vi "Analog Output - 1 Channel - 1 Sample.vi"() -> ()   [LabVIEW 2019]
uses:
  <vilib>/myRIO/Instrument Drivers/Onboard IO/AO/typedefs/AO Reference.ctl
  <vilib>/myRIO/Common/Instrument Driver Framework/Utilities/typedefs/myRIO Generic Hardware Reference.ctl
  <vilib>/myRIO/Common/Instrument Driver Framework/Utilities/typedefs/Hardware Version Enum.ctl
  <vilib>/myRIO/Common/Instrument Driver Framework/Utilities/typedefs/myRIO v1.0 Reference.ctl
  <vilib>/myRIO/Common/Instrument Driver Framework/Utilities/typedefs/Generic FPGA Reference.ctl
  <vilib>/myRIO/Common/Instrument Driver Framework/myRIO v1.0/AO/typedefs/AO Channels List.ctl
  <vilib>/myRIO/Common/Instrument Driver Framework/myRIO v1.0/AO/typedefs/AO Channels Enum.ctl
  <vilib>/myRIO/Common/Instrument Driver Framework/Utilities/typedefs/Analog Scaling Constants List.ctl
  <vilib>/myRIO/Common/Instrument Driver Framework/Utilities/typedefs/Analog Scaling Constants.ctl
  <vilib>/userdefined/High Color/nirio_resource_hc.ctl
  <vilib>/myRIO/Common/Instrument Driver Framework/Utilities/vis/Is FPGA Ref Available.vi
  <vilib>/myRIO/Common/Instrument Driver Framework/ELVIS III v1.0/AO/vis/ELVIS III v1.1 Open AO.vi
  <vilib>/myRIO/Instrument Drivers/Onboard IO/AO/vis/Write.vi
  <vilib>/myRIO/Common/Instrument Driver Framework/Utilities/vis/Validate Channels.vi
  <vilib>/myRIO/Common/Instrument Driver Framework/ELVIS III v1.0/AO/vis/ELVIS III v1.0 Reserve AO.vi
  <vilib>/myRIO/Common/Instrument Driver Framework/myRIO v1.0/UART/vis/myRIO v1.0 Close UART.vi
  <vilib>/myRIO/Common/Instrument Driver Framework/ELVIS III v1.0/AO/vis/ELVIS III v1.0 Build MUX Configuration AO.vi
  <vilib>/Utility/VariantDataType/GetNumericInfo.vi
  <vilib>/Utility/error.llb/Error Cluster From Error Code.vi
  <vilib>/myRIO/Common/Instrument Driver Framework/ELVIS III v1.0/ELVIS III v1.1 Open.vi
  <vilib>/myRIO/Common/Instrument Driver Framework/ELVIS III v1.0/Resource Manager/vis/ELVIS III v1.0 Reserve Channel List.vi
  <vilib>/myRIO/Common/Instrument Driver Framework/myRIO v1.0/myRIO v1.0 Close.vi
  <vilib>/myRIO/Common/Instrument Driver Framework/ELVIS III v1.0/AO/vis/ELVIS III v1.0 Write AO.vi
  <vilib>/myRIO/Common/Instrument Driver Framework/Utilities/vis/FPGA Ref Manager.vi
  <vilib>/myRIO/Common/Instrument Driver Framework/ELVIS III v1.0/ELVIS III v1.0 Reset FPGA.vi
  <vilib>/myRIO/Common/Instrument Driver Framework/myRIO v1.0/IRQ/vis/myRIO v1.0 IRQ Info FGV.vi
  <vilib>/myRIO/Common/Instrument Driver Framework/myRIO v1.0/IRQ/vis/myRIO v1.0 Timer IRQ Info FGV.vi
  <vilib>/myRIO/Common/Instrument Driver Framework/myRIO v1.0/IRQ/vis/myRIO v1.0 ISR Agent.vi
  <vilib>/myRIO/Instrument Drivers/Utilities/vis/Reset Index.vi
  <vilib>/myRIO/Common/Instrument Driver Framework/myRIO v1.0/Resource Manager/vis/myRIO v1.0 Block Write Resource Manager.vi
  <vilib>/myRIO/Express VI/Onboard IO/AO/AO Express VI.xnode
  <vilib>/myRIO/Instrument Drivers/Onboard IO/AO/vis/myRIO AO Open.xnode
  <vilib>/myRIO/Instrument Drivers/Utilities/Utilities.lvlib
  <vilib>/myRIO/Instrument Drivers/Onboard IO/AO/AO.lvlib
panel:
  in  "A/AO0 (V)":dbl min=-10.0 max=10.0 step=0.1
  in  "Stop":bool
  # "ELVIS III Control IO"
  # "模拟输出单通道"
  # "Overview: Generates a voltage value on Bank A, Channel AO0 (A/AO0).\nInstructions:\n1. Select a voltage value below.\n2. Connect A/AO0 to the positive lead of the load, and connect AGND to the negative lead of the load. AGND is the ground reference terminal for analog output channels.\n3. Run the VI.\nNote: You can change the AO value while the VI is running."
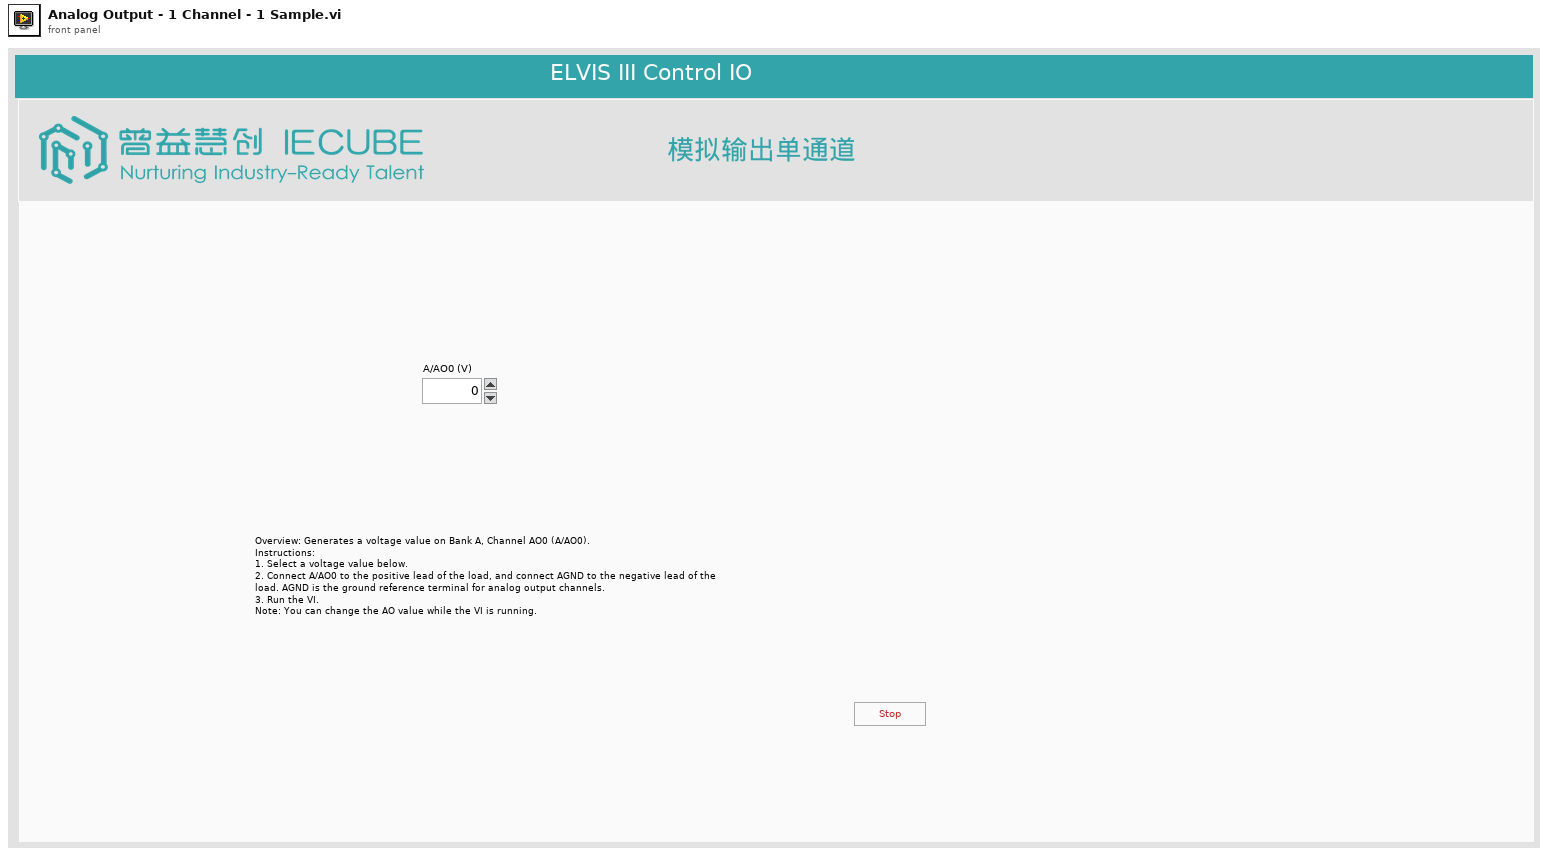
[diagram p1: front panel]
types:
  T1 = typedef "AO.lvlib/AO Reference.ctl" = cluster{"myRIO Reference":T2, "AO Channel List":T6, "AO Scaling Constant List":T8}
  T2 = typedef "myRIO Generic Hardware Reference.ctl" = cluster{"myRIO Model":T3, "myRIO Hardware Reference":T4}
  T3 = typedef "Hardware Version Enum.ctl" = enum16{"Unknown", "myRIO-1900", "myRIO-1950", "roboRIO", "NI ELVIS RIO CM", "ELVIS III"}
  T4 = typedef "myRIO v1.0 Reference.ctl" = cluster{"Generic FPGA Reference":T5, "Allow multiple opens":bool}
  T5 = typedef "Generic FPGA Reference.ctl" = refnum<k20>
  T6 = typedef "AO Channels List.ctl" = T7[]
  T7 = typedef "AO Channels Enum.ctl" = enum16{"Not Connected", "AudioOut/Left", "AudioOut/Right", "C/AO0", "C/AO1", "A/AO0", "A/AO1", "B/AO0", "B/AO1"}
  T8 = typedef "Analog Scaling Constants List.ctl" = T9[]
  T9 = typedef "Analog Scaling Constants.ctl" = cluster{"LSB Weight (Volts)":dbl, "Offset (Volts)":dbl, "Signed?":bool}
  T10 = typedef "nirio_resource_hc.ctl" = tag
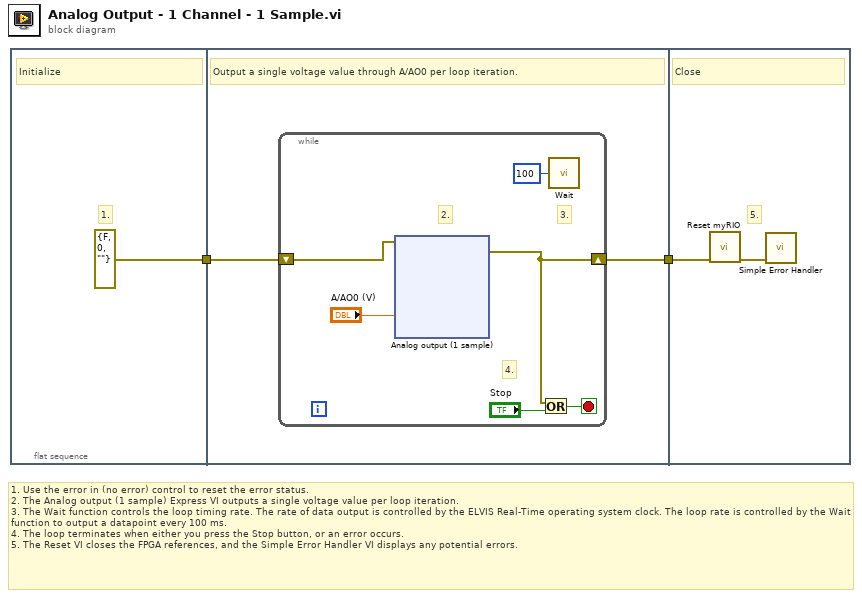
[diagram p0: block diagram]
diagram:
  # "1. Use the error in (no error) control to reset the error status. \n2. The Analog output (1 sample) Express VI outputs a single voltage value per loop iteration.\n3. The Wait function controls the loop timing rate. The rate of data output is controlled by the ELVIS Real-Time operating system clock. The loop rate is controlled by the Wait function to output a datapoint every 100 ms.\n4. The loop terminates when either you press the Stop button, or an error occurs.\n5. The Reset VI closes the FPGA references, and the Simple Error Handler VI displays any potential errors."
  n1 = flat-sequence {
    tunnel: [errorcluster {"status"=FALSE, "code"=0, "source"=""} ("Error In")] -> w1
    tunnel: [w5] -> w2
    tunnel: w1 -> [w4]
    tunnel: w2 -> [w50]
    frame #0 {
      # "1."
      # "Initialize"
    }
    frame #1 {
      # "Output a single voltage value through A/AO0 per loop iteration."
      n2 = while {
        shift-right: [w10] -> w5
        shift-left: w4 -> [w9]
        stop <- w11 stop-if-true
        # "4."
        # "3."
        # "2."
        n3 = xnode "Analog output (1 sample)"("A/AO0"="A/AO0 (V)", "error in (no error)"=w9) -> ("error out"=w10:errorcluster)
        n4 = Or(x=w10, y="Stop") -> (x .or. y?=w11:bool)
        n5 = call "Wait"("Count(mSec)"=u32 100) -> ()  [unwired: 1 out]
      }
    }
    frame #2 {
      # "5."
      # "Close"
      n6 = call <vilib>:"Reset myRIO.vi"("error in (no error)"=w50) -> ("error out"=w49:errorcluster)  [unwired: 10 in]
      n7 = call <vilib>:"Simple Error Handler.vi"("error in (no error)"=w49) -> ()  [unwired: 4 in, 5 out]
    }
  }
